vi "Prepare Left and Right Menus Strings.vi"(8 "error in (no error)":errorcluster, 10 "Right Menu ref":refnum<vi>, 11 "Left Menu ref":refnum<vi>) -> (0 "error out":errorcluster)   [LabVIEW 2020, in "ATM.lvlib"]
uses:
  ATM.lvlib
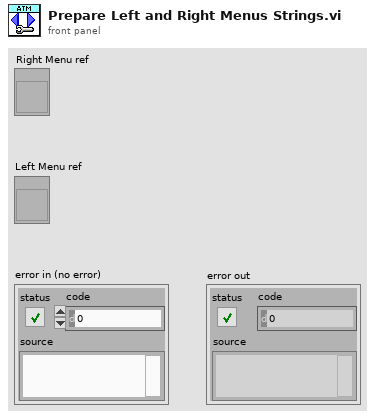
[diagram p1: front panel]
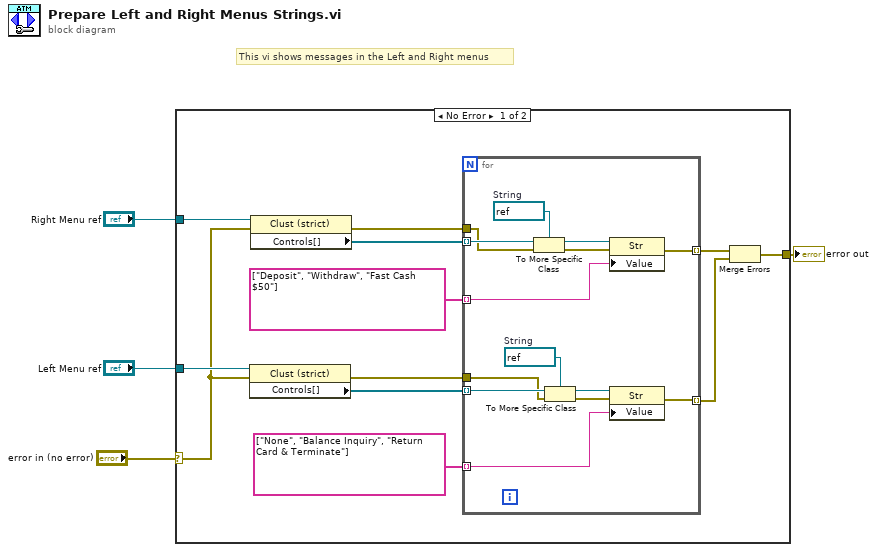
[diagram p0: block diagram]
diagram:
  # "This vi shows messages in the Left and Right menus"
  n1 = case shown="No Error" "error in (no error)" {
    selector: "error in (no error)" -> [w10 w31]
    tunnel: "Right Menu ref" -> [w16 _]
    tunnel: "Left Menu ref" -> [w15 _]
    tunnel: [w5 w31] -> w1
    frame No Error {
      n2 = property class="Clust (strict)"(reference=w15, error in=w10) -> (error out=w8:errorcluster, "Controls[]"=w13:refnum<vi>[])  [unwired: 1 out]
      n3 = property class="Clust (strict)"(reference=w16, error in=w10) -> (error out=w9:errorcluster, "Controls[]"=w14:refnum<vi>[])  [unwired: 1 out]
      n4 = for {
        tunnel: w14 -> [w30] mode=indexing
        tunnel: w13 -> [w25] mode=indexing
        tunnel: string[] ["None", "Balance Inquiry", "Return Card & Terminate"] -> [w23] mode=indexing
        tunnel: string[] ["Deposit", "Withdraw", "Fast Cash $50"] -> [w27] mode=indexing
        tunnel: w9 -> [w22]
        tunnel: [w20] -> w7 mode=indexing
        tunnel: [w19] -> w6 mode=indexing
        tunnel: w8 -> [w17]
        w26 = refnum<vi> refnum  # String
        w28 = refnum<vi> refnum  # String
        n5 = To More Specific Class(target class=w28, reference=w30, error in=w22) -> (specific class reference=w29:refnum<vi>, error out=w21:errorcluster)
        n6 = To More Specific Class(target class=w26, reference=w25, error in=w17) -> (specific class reference=w24:refnum<vi>, error out=w18:errorcluster)
        n7 = property class="Str"(reference=w29, error in=w21, "Value"=w27) -> (error out=w20:errorcluster)  [unwired: 1 out]
        n8 = property class="Str"(reference=w24, error in=w18, "Value"=w23) -> (error out=w19:errorcluster)  [unwired: 1 out]
      }
      n9 = Merge Errors(w7, w6) -> (w5:errorcluster)
    }
    frame Error {
    }
  }
  "error out" <- w1
